vi "ui_DataLog Query Tag Creation Parameters.vi"(7 "default config":T1 {"logging parameters" format="%.2e"; "precision" items=["0", "1", "2", "3", "4", "5", "6", "7", "8", "9", "10", "11", "12", "13", "14", "15", "16", "17"]; "limit delay" format="%.2e"; "deadband" format="%.2e"}) -> (3 "initial value out":dbl format="%.2f", 4 "OKed?":bool, 8 "info out":T1 {"logging parameters" format="%.2e"; "precision" items=["0", "1", "2", "3", "4", "5", "6", "7", "8", "9", "10", "11", "12", "13", "14", "15", "16", "17"]; "limit delay" format="%.2e"; "deadband" format="%.2e"}, 15 "initial string out":string)   [LabVIEW 2012]
doc: "This dialog queries for the subset of tag parameters that can only be set once, when the tag is created."
uses:
  typedefs/t_DataLog Temporal Types.ctl
  typedefs/t_DataLog Value Types.ctl
  typedefs/clusters/t_DataLog Tag Config.ctl
  typedefs/t_DataLog Numerical Format.ctl
  typedefs/t_DataLog Logging Algorithms.ctl
  typedefs/t_DataLog Query Tag Creation Parameters States.ctl
  glb_DataLog MCVD.vi
panel:
  in  "initial string":string
  in  "initial number":dbl format="%.4e"
  in  "unit":string
  in  "value type":T3
  in  "temporal type":T2
  in  "cancel":bool
  in  "OK":bool
  # "Once the tag has been created, these tag\nparameters can no longer be modified."
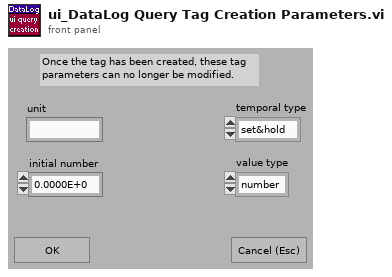
[diagram p1: front panel]
types:
  T1 = typedef "t_DataLog Tag Config.ctl" = cluster{"name":string, "unit":string, "temporal":T2, "value":T3, "index":i32, "capacity":i32, "is meta?":bool, "mincapacity":i32, "deadband":dbl, "limit delay":dbl, "format":T4, "precision":u8, "undefine":bool, "update":bool, "update period":u16, "expression":string, "description":string, "logging algorithm":T5, "logging parameters":dbl[]}
  T2 = typedef "t_DataLog Temporal Types.ctl" = enum16{"set&hold", "sample", "event"}
  T3 = typedef "t_DataLog Value Types.ctl" = enum16{"number", "string"}
  T4 = typedef "t_DataLog Numerical Format.ctl" = enum8{"fractional", "exponential", "engineering"}
  T5 = typedef "t_DataLog Logging Algorithms.ctl" = enum16{"nothing", "changes", "everything", "every Nth", "time threshold", "value threshold + prior", "t or v threshold", "t or v threshold + prior"}
  T6 = typedef "t_DataLog Query Tag Creation Parameters States.ctl" = enum16{"empty queue", "ablement", "initialize", "stop"}
  T7 = typedef "eventvkey.ctl" = enum16{"ASCII", "Enter", "Return", "Shift", "Ctrl", "Alt", "Cmd", "Opt", "Caps", "NumLock", "Clear", "Break", "Up", "Down", "Left", "Right", "Insert", "Delete", "Home", "End", "PageUp", "PageDown", "Escape", "Help", "Pause", "ScrollLock", "F1", "F2", "F3", "F4", "F5", "F6", "F7", "F8", "F9", "F10", "F11", "F12", "F13", "F14", "F15", "F16", "F17", "F18", "F19", "F20", "F21", "F22", "F23", "F24", "Play", "VolumeUp", "VolumeDown", "Mute", "Two Byte Char"}
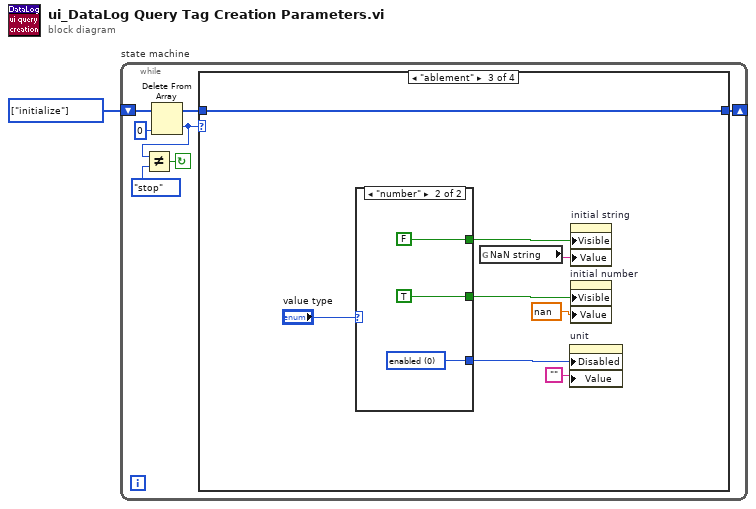
[diagram p0: block diagram]
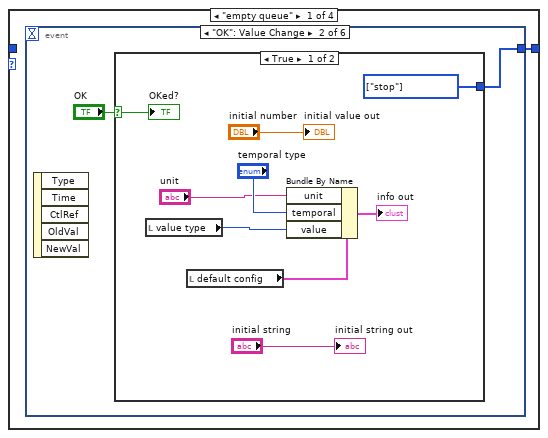
[diagram p2: hidden frame]
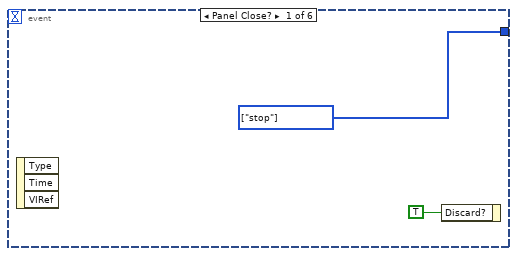
[diagram p3: hidden frame]
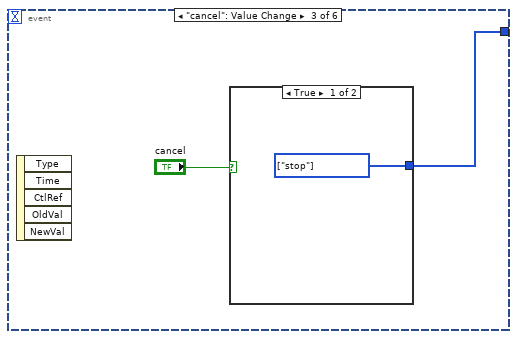
[diagram p5: hidden frame]
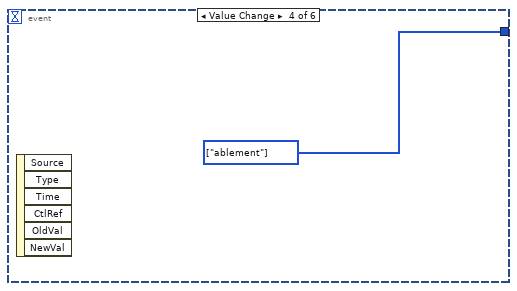
[diagram p7: hidden frame]
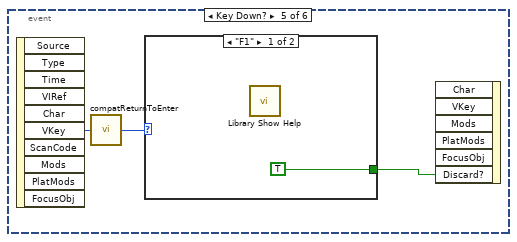
[diagram p8: hidden frame]
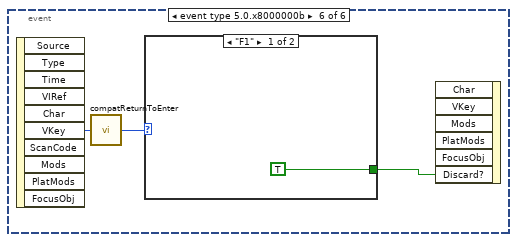
[diagram p10: hidden frame]
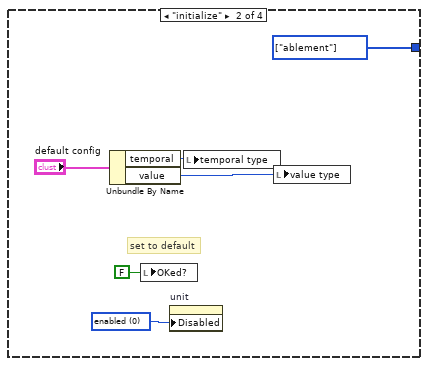
[diagram p12: hidden frame]
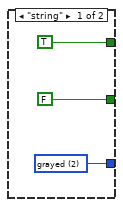
[diagram p13: hidden frame]
diagram:
  w1 = T6[] [enum."initialize"] items=["empty queue", "ablement", "initialize", "stop"] ("Array Constant")
  n1 = while "state machine" {
    shift-left: w1 -> [w5]
    shift-right: [w8] -> _
    stop <- w7 continue-if-true
    n2 = Delete From Array(array=w5, index=0) -> (deleted portion=w3:T6, array with subset deleted=w4:T6[])  [unwired: 1 in]
    n3 = Not Equal?(x=w3, y=t_DataLog_Query_Tag_Creation_Parameters_States."stop" ("states")) -> (x != y?=w7:bool)
    n4 = case "Case" shown="\"ablement\"" w3 {
      tunnel: [w9 w36 w48 w55] -> w8
      tunnel: w4 -> [_ _ w48 w55]
      frame "empty queue" {
        n5 = event shown="[1] \"OK\": Value Change" {
          selector: _ -> [_ _ _ _ _ _]
          dyn-events: _ -> [_ _ _ _ _ _]
          timeout: _ -> [_ _ _ _ _ _]
          tunnel: [w11 w13 w24 w26 _ _] -> w9
          event Panel Close? {
            w11 = T6[] [enum."stop"] items=["empty queue", "ablement", "initialize", "stop"] ("Array Constant")
            n6 = event-data() -> ()  [unwired: 1 in, 3 out]
            n7 = event-data("Discard?"=TRUE) -> ()  [unwired: 1 in, 1 out]
          }
          event "OK": Value Change {
            n8 = event-data() -> ()  [unwired: 1 in, 5 out]
            n9 = case shown="True" "OK" {
              selector: "OK" -> [w21 _]
              tunnel: [w22 _] -> w13
              frame True {
                w22 = T6[] [enum."stop"] items=["empty queue", "ablement", "initialize", "stop"] ("Array Constant")
                n10 = local read "value type"() -> (w14:T3)
                n11 = local read "default config"() -> (w20:T1)
                n12 = Bundle By Name(cluster=w20, "unit"="unit", "temporal"="temporal type", "value"=w14) -> (→"info out":T1)
                "OKed?" <- w21
                "initial value out" <- "initial number"
                "initial string out" <- "initial string"
              }
              frame False {
              }
            }
          }
          event "cancel": Value Change {
            n13 = event-data() -> ()  [unwired: 1 in, 5 out]
            n14 = case shown="True" "cancel" {
              tunnel: [w25 _] -> w24
              frame True {
                w25 = T6[] [enum."stop"] items=["empty queue", "ablement", "initialize", "stop"] ("Array Constant")
              }
              frame False {
              }
            }
          }
          event Value Change {
            w26 = T6[] [enum."ablement"] items=["empty queue", "ablement", "initialize", "stop"] ("Array Constant")
            n15 = event-data() -> ()  [unwired: 1 in, 6 out]
          }
          event Key Down? {
            n16 = event-data() -> ("VKey"=w27:T7)  [unwired: 1 in, 9 out]
            n17 = call <vilib>:"compatReturnToEnter.vi"("VKey"=w27) -> ("VKey"=w29:T7)
            n18 = case shown="\"F1\"" w29 {
              tunnel: [TRUE _] -> w28
              frame "F1" {
                n19 = call "Library Show Help.vi"() -> ()  [unwired: 1 in]
              }
              frame Default {
              }
            }
            n20 = event-data("Discard?"=w28) -> ()  [unwired: 6 in, 1 out]
          }
          event event type 5.0.x8000000b {
            n21 = event-data() -> ("VKey"=w31:T7)  [unwired: 1 in, 9 out]
            n22 = call <vilib>:"compatReturnToEnter.vi"("VKey"=w31) -> ("VKey"=w33:T7)
            n23 = case shown="\"F1\"" w33 {
              tunnel: [TRUE _] -> w32
              frame "F1" {
              }
              frame Default {
              }
            }
            n24 = event-data("Discard?"=w32) -> ()  [unwired: 6 in, 1 out]
          }
        }
      }
      frame "initialize" {
        w36 = T6[] [enum."ablement"] items=["empty queue", "ablement", "initialize", "stop"] ("Array Constant")
        w37 = u8 0 items=["enabled", "disabled", "grayed"] ("disabled state")
        # "set to default"
        n25 = Unbundle By Name("default config") -> ("temporal"=w39:T2, "value"=w35:T3)
        n26 = local write "OKed?"(FALSE ("OKed?")) -> ()
        n27 = property on="unit" class="Str"("Disabled"=w37) -> ()  [unwired: 2 in, 2 out]
        n28 = local write "temporal type"(w39) -> ()
        n29 = local write "value type"(w35) -> ()
      }
      frame "ablement" {
        n30 = case shown="\"number\"" "value type" {
          tunnel: [w51 w54] -> w46
          tunnel: [TRUE FALSE] -> w44
          tunnel: [FALSE TRUE] -> w43
          frame "string" {
            w51 = u8 2 items=["enabled", "disabled", "grayed"] ("disabled state")
          }
          frame "number" {
            w54 = u8 0 items=["enabled", "disabled", "grayed"] ("disabled state")
          }
        }
        n31 = global read "glb_DataLog MCVD.vi" "NaN string"() -> (w42:string)
        n32 = property on="unit" class="Str"("Disabled"=w46, "Value"="") -> ()  [unwired: 2 in, 2 out]
        n33 = property on="initial string" class="Str"("Visible"=w44, "Value"=w42) -> ()  [unwired: 2 in, 2 out]
        n34 = property on="initial number" class="DigNum (strict)"("Visible"=w43, "Value"=nan ("initial value")) -> ()  [unwired: 2 in, 2 out]
      }
      frame "stop" {
      }
    }
  }
